vi "poly_lock_fp_updates_lock_fp_ref.vi"(8 "error in":errorcluster, 9 "fp ref":refnum<vi>) -> (0 "error out":errorcluster)   [LabVIEW 2015]
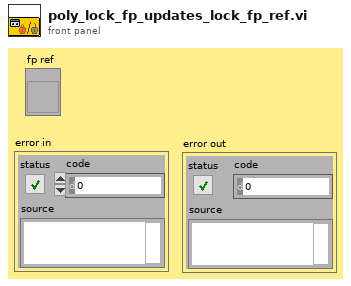
[diagram p1: front panel]
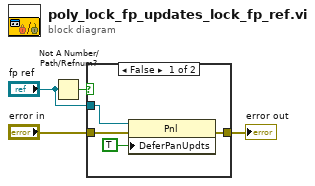
[diagram p0: block diagram]
diagram:
  n1 = Not A Number/Path/Refnum?(number/path/refnum="fp ref") -> (NaN/Path/Refnum?=w1:bool)
  n2 = case shown="False" w1 {
    tunnel: [w7 w9] -> w4
    tunnel: "fp ref" -> [w6 _]
    tunnel: "error in" -> [w5 w9]
    frame False {
      n3 = property class="Pnl"(reference=w6, error in=w5, "DeferPanUpdts"=TRUE) -> (error out=w7:errorcluster)  [unwired: 1 out]
    }
    frame True {
    }
  }
  "error out" <- w4
